vi "bpms.vi"() -> ()   [LabVIEW 2015]
uses:
  <vilib>/Instr/_visa.llb/VISA Configure Serial Port (Instr).vi
panel:
  out "String":string
  in  "VISA resource name":refnum<visa-resource-name>
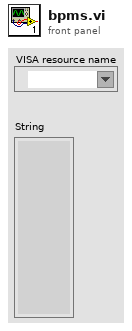
[diagram p1: front panel]
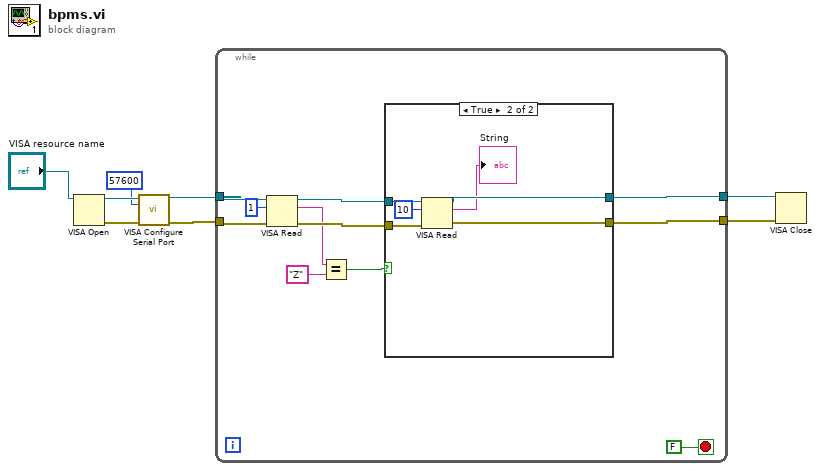
[diagram p0: block diagram]
diagram:
  n1 = VISA Open(VISA resource name="VISA resource name") -> (VISA resource name=w7:refnum<visa-resource-name>, error out=w6:errorcluster)  [unwired: 4 in]
  n2 = call-poly "VISA Configure Serial Port"("VISA resource name"=w7, "baud rate (9600)"=u32 57600, "error in (no error)"=w6) -> ("VISA resource name out"=w4:refnum<visa-resource-name>, "error out"=w3:errorcluster)  [unwired: 11 in]
  n3 = while {
    tunnel: w4 -> [w17]
    tunnel: w3 -> [w16]
    tunnel: [w13] -> w2
    tunnel: [w12] -> w1
    stop <- FALSE stop-if-true
    n4 = VISA Read(VISA resource name=w17, byte count=u32 1, error in (no error)=w16) -> (VISA resource name out=w15:refnum<visa-resource-name>, read buffer=w10:string, error out=w14:errorcluster)  [unwired: 1 out]
    n5 = Equal?(x=w10, y="Z") -> (x = y?=w11:bool)
    n6 = case shown="True" w11 {
      tunnel: w15 -> [w21 w26]
      tunnel: w14 -> [w20 w25]
      tunnel: [w21 w24] -> w13
      tunnel: [w20 w23] -> w12
      frame False {
      }
      frame True {
        n7 = VISA Read(VISA resource name=w26, byte count=u32 10, error in (no error)=w25) -> (VISA resource name out=w24:refnum<visa-resource-name>, read buffer=→"String":string, error out=w23:errorcluster)  [unwired: 1 out]
      }
    }
  }
  n8 = VISA Close(VISA resource name=w2, error in (no error)=w1) -> ()  [unwired: 1 out]
